vi "appendElement.vi"(7 "Document in":refnum<class "xwpfDocument.lvclass">, 8 "error in (no error)":errorcluster, 11 "xwpfParagraph in":refnum<class "xwpfParagraph.lvclass">) -> (0 "error out":errorcluster, 3 "xwpfParagraph out":refnum<class "xwpfParagraph.lvclass">, 5 "Document out":refnum<class "xwpfDocument.lvclass">)   [LabVIEW 2017, in "Word_Specific.lvlib" / "xwpfParagraph.lvclass"]
uses:
  xwpfParagraph.lvclass
  xwpfDocument/xwpfDocument.lvclass
  xwpfParagraph.lvclass/xwpfParagraph.ctl
  xwpfRun/xwpfRun.lvclass/xwpfRun.ctl
  xwpfRun/Get Text.vi
  xwpfRun/Get Style.vi
  Get Runs.vi
  Styles/Style/Style.lvclass
  xwpfRun/xwpfRun.lvclass
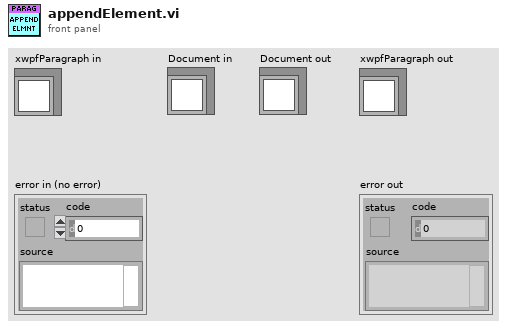
[diagram p1: front panel]
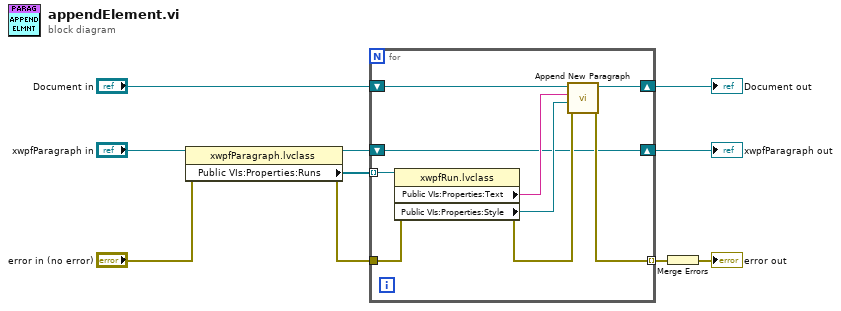
[diagram p0: block diagram]
diagram:
  n1 = property class="xwpfParagraph.lvclass"(reference="xwpfParagraph in", error in="error in (no error)") -> (reference out=w2:refnum<class "xwpfParagraph.lvclass">, error out=w8:errorcluster, "Public VIs:Properties:Runs"=w9:refnum<class "xwpfRun.lvclass">[])
  n2 = for {
    tunnel: w9 -> [w19] mode=indexing
    tunnel: w8 -> [w18]
    tunnel: [w13] -> w4 mode=indexing
    shift-right: [w12] -> w6
    shift-left: "Document in" -> [w17]
    shift-right: [w11] -> w1
    shift-left: w2 -> [w11]
    n3 = property class="xwpfRun.lvclass"(reference=w19, error in=w18) -> (error out=w14:errorcluster, "Public VIs:Properties:Text"=w16:string, "Public VIs:Properties:Style"=w15:refnum<class "Style.lvclass">)  [unwired: 1 out]
    n4 = call "Append New Paragraph.vi"("error in (no error)"=w14, "Paragraph.Style"=w15, "Paragraph.Text"=w16, "xwpfDocument in"=w17) -> ("error out"=w13:errorcluster, "xwpfDocument out"=w12:refnum<class "xwpfDocument.lvclass">)  [unwired: 6 in]
  }
  "xwpfParagraph out" <- w1
  "Document out" <- w6
  n5 = Merge Errors(w4) -> (→"error out":errorcluster)
